vi "Array, Initialize Diagonal, DBL.vi"(1 "dimension":i32[](array[numeric])=[3, 3], 2 "diagonal":dbl=1.0 format="%.1f", 3 "fill":dbl format="%.1f") -> (0 "new array":dbl[][](array[numeric]) format="%.1g")   [LabVIEW 2010]
doc: "This function creates an array with element and diagonal fill options."
uses:
  <vilib>/Analysis/Matrix/Numeric/Conversions/Array To Matrix - RA2.vi
  <vilib>/Analysis/Matrix/Numeric/Conversions/Matrix To Array - RM.vi
  <vilib>/Analysis/Matrix/NI_Matrix.lvlib
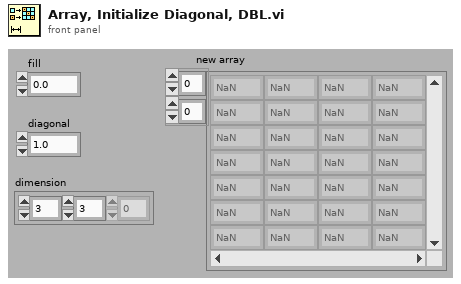
[diagram p1: front panel]
types:
  T1 = typedef "NI_Matrix.lvlib/RealMatrix.ctl" = dbl[][]
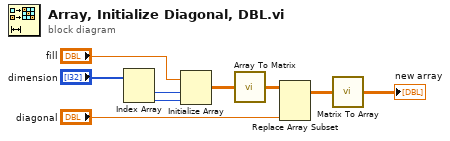
[diagram p0: block diagram]
diagram:
  n1 = Index Array(array="dimension") -> (element #1=w6:i32, element #2=w7:i32)  [unwired: 2 in]
  n2 = Initialize Array("fill", w6, w7) -> (w4:dbl[][])
  n3 = call-poly <vilib>:"Array To Matrix.vi"("Real 2D Array"=w4) -> ("Real Matrix"=w9:T1)
  n4 = Replace Array Subset(array=w9, new element="diagonal") -> (w8:T1)  [unwired: 2 in]
  n5 = call-poly <vilib>:"Matrix To Array.vi"("Real Matrix"=w8) -> ("Real 2D Array"=→"new array":dbl[][])
